vi "gitMonitor.vi"() -> ()   [LabVIEW 2023, in "gitTools.lvlib"]
uses:
  gitTools.lvlib
  repoDetails.ctl
panel:
  out "repos":T1[](array[typedef])
  in  "Monitoring Folder":path
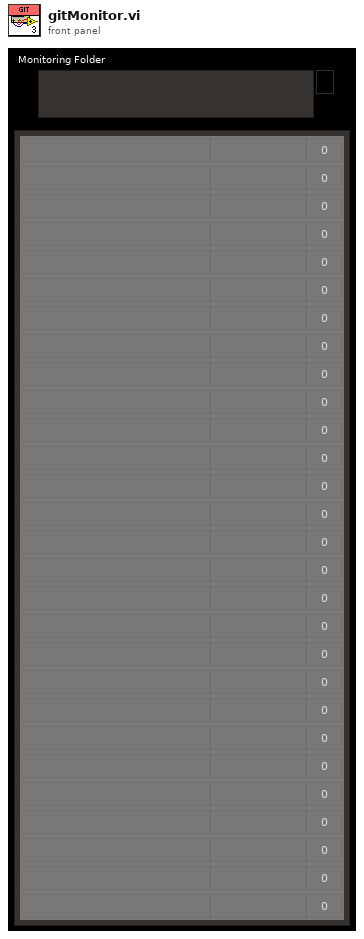
[diagram p1: front panel]
types:
  T1 = typedef "gitTools.lvlib/repoDetails.ctl" = cluster{"Repo Folder":string, "Branch":string, "changes":u32}
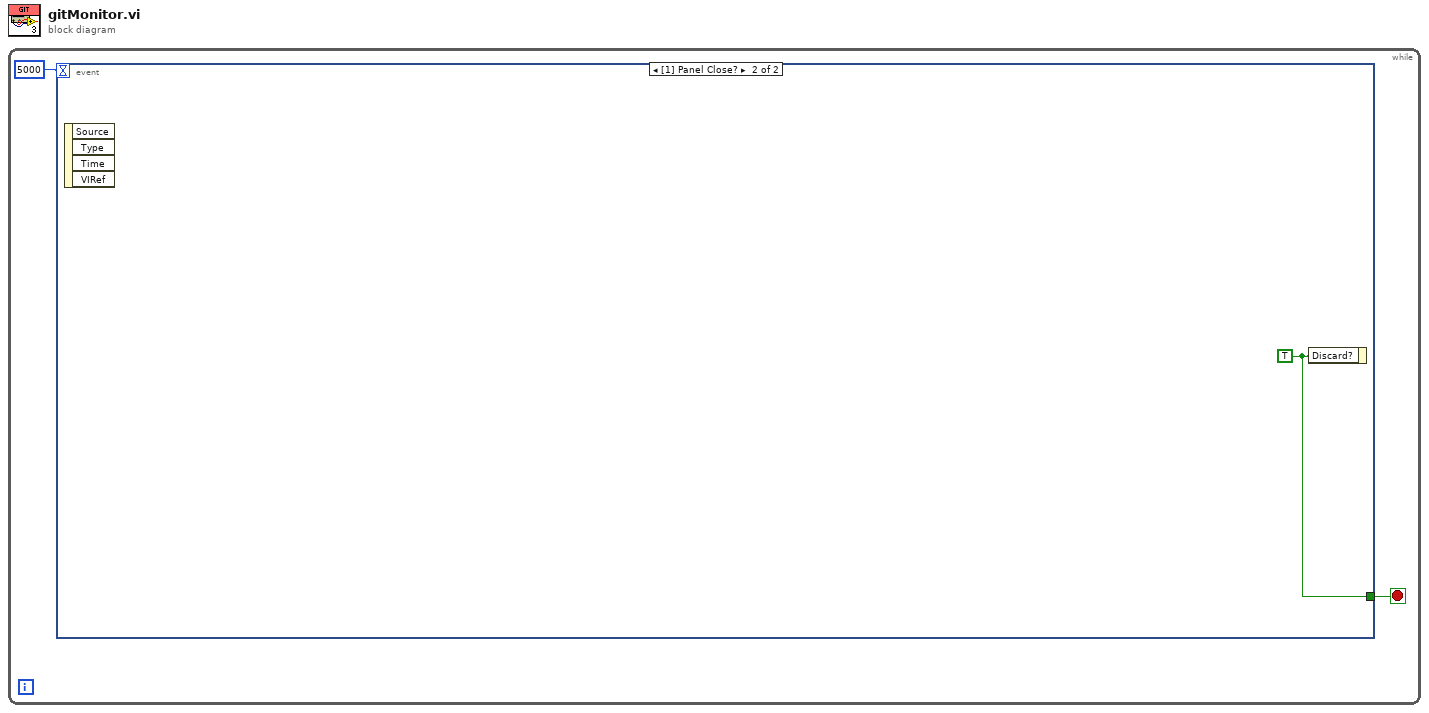
[diagram p0: block diagram]
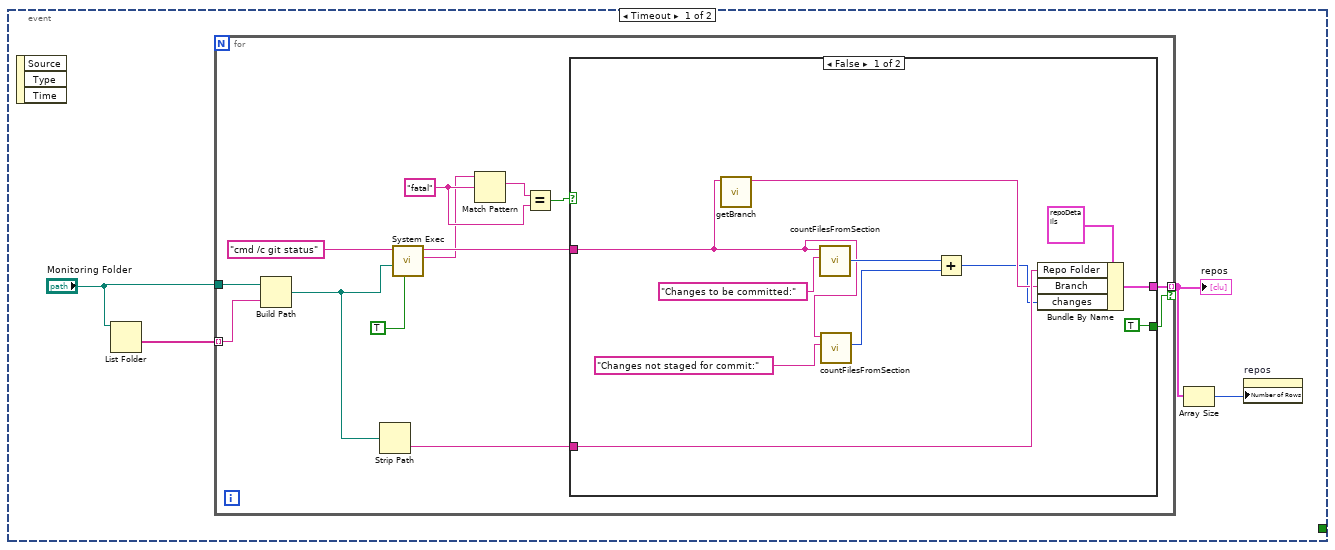
[diagram p2: hidden frame]
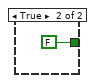
[diagram p3: hidden frame]
diagram:
  n1 = while {
    stop <- w1 stop-if-true
    n2 = event shown="[1] Panel Close?" {
      selector: _ -> [_ _]
      dyn-events: _ -> [_ _]
      timeout: 5000 -> [_ _]
      tunnel: [_ w32] -> w1
      event Timeout {
        n3 = event-data() -> ()  [unwired: 1 in, 3 out]
        n4 = List Folder(path="Monitoring Folder") -> (folder names=w6:string[])  [unwired: 3 in, 3 out]
        n5 = for {
          tunnel: [w16] -> w4 mode=indexing if=w8
          tunnel: w6 -> [w14] mode=indexing
          tunnel: "Monitoring Folder" -> [w15]
          w10 = "fatal" ("regular expression")
          n6 = Build Path(base path=w15, name or relative path=w14) -> (appended path=w13:path)
          n7 = Strip Path(path=w13) -> (name=w17:string)  [unwired: 1 out]
          n8 = call <vilib>:"System Exec.vi"("run minimized? (F)"=TRUE, "working directory"=w13, "command line"="cmd /c git status") -> ("standard error"=w7:string, "standard output"=w12:string)  [unwired: 5 in, 2 out]
          n9 = Match Pattern(string=w7, regular expression=w10) -> (match substring=w11:string)  [unwired: 1 in, 3 out]
          n10 = Equal?(x=w11, y=w10) -> (x = y?=w9:bool)
          n11 = case shown="False" w9 {
            tunnel: w17 -> [w29 _]
            tunnel: [w28 _] -> w16
            tunnel: w12 -> [w21 _]
            tunnel: [TRUE FALSE] -> w8
            frame False {
              n12 = call "getBranch.vi"("gitStatusResponse"=w21) -> ("branch"=w27:string)  [unwired: 10 in]
              n13 = call "countFilesFromSection.vi"("sectionToCountFiles"="Changes to be committed:" ("regular expression"), "text"=w21) -> ("count"=w24:u32)  [unwired: 9 in]
              n14 = call "countFilesFromSection.vi"("sectionToCountFiles"="Changes not staged for commit:", "text"=w21) -> ("count"=w23:u32)  [unwired: 9 in]
              n15 = Add(x=w24, y=w23) -> (x+y=w22:u32)
              n16 = Bundle By Name(cluster=T1 {"Repo Folder"="constellation-polaris-webserver", "Branch"="development", "changes"=0} ("repoDetails"), "Repo Folder"=w29, "Branch"=w27, "changes"=w22) -> (w28:T1)
            }
            frame True {
            }
          }
        }
        "repos" <- w4
        n17 = Array Size(array=w4) -> (size(s)=w3:i32)
        n18 = property on="repos" class="Arr (strict)"("Number of Rows"=w3) -> ()  [unwired: 2 in, 2 out]
      }
      event Panel Close? {
        w32 = TRUE ("Discard?")
        n19 = event-data() -> ()  [unwired: 1 in, 4 out]
        n20 = event-data("Discard?"=w32) -> ()  [unwired: 1 in, 1 out]
      }
    }
  }
